vi "Read Credentials.vi"(8 "error in (no error)":errorcluster, 11 "AWS Core in":refnum<class "AWS Core.lvclass">) -> (0 "error out":errorcluster, 2 "Credentials":T1, 3 "AWS Core out":refnum<class "AWS Core.lvclass">)   [LabVIEW 2015, in "AWS Core.lvlib" / "AWS Core.lvclass"]
uses:
  AWS Core.lvclass
  AWS Credentials.ctl
  AWS Core.lvclass/AWS Core.ctl
  AWS Core.lvlib
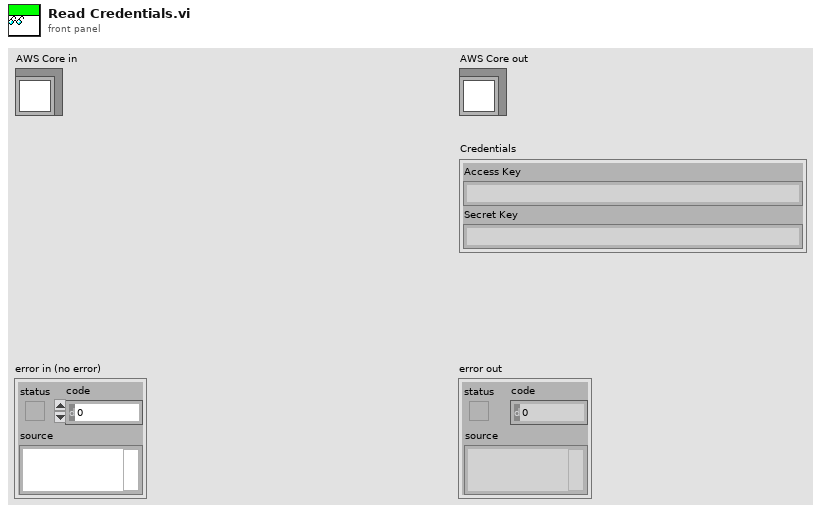
[diagram p1: front panel]
types:
  T1 = typedef "AWS Core.lvlib/AWS Credentials.ctl" = cluster{"Access Key":string, "Secret Key":string}
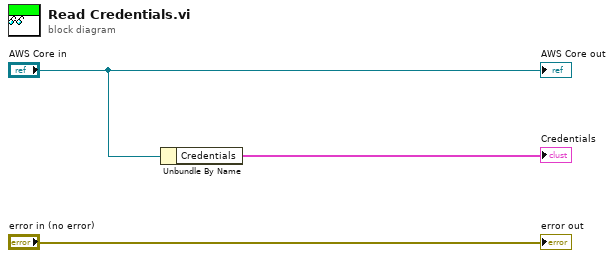
[diagram p0: block diagram]
diagram:
  n1 = Unbundle By Name("AWS Core in") -> ("Credentials"=→"Credentials":T1)
  "error out" <- "error in (no error)"
  "AWS Core out" <- "AWS Core in"
